vi "RTM - Import from XML.vi"(8 "error in (no error)":errorcluster, 11 "Node Ptr":u64 format="%.0x") -> (0 "error out":errorcluster)   [LabVIEW 2019, in "UDP-Custom-Device System Explorer.lvlib"]
uses:
  UDP-Custom-Device System Explorer.lvlib
panel:
  in  "Tag":string
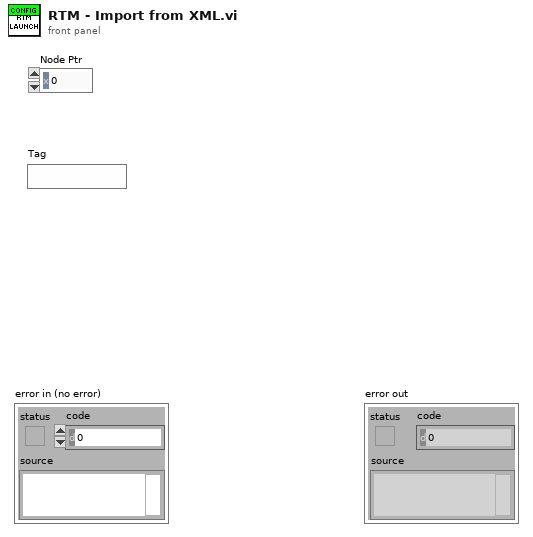
[diagram p1: front panel]
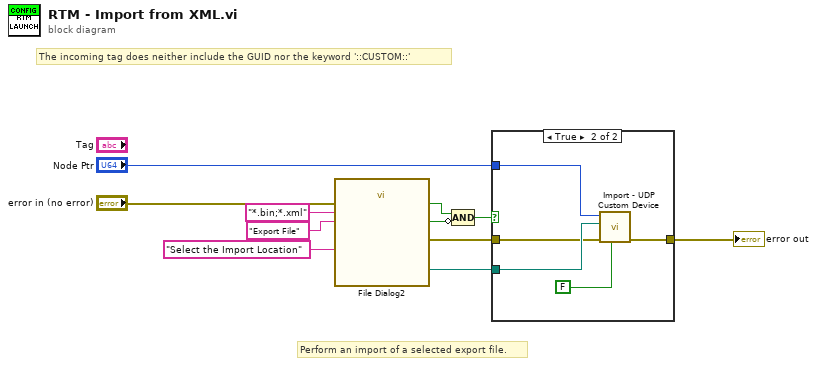
[diagram p0: block diagram]
diagram:
  # "Perform an import of a selected export file."
  # "The incoming tag does neither include the GUID nor the keyword '::CUSTOM::'"
  n1 = call "File Dialog2"("prompt"="Select the Import Location", "error in"="error in (no error)", "pattern (all files)"="*.bin;*.xml", "pattern label"="Export File") -> ("selected path"=w7:path, "exists"=w5:bool, "cancelled"=w4:bool, "error out"=w6:errorcluster)  [unwired: 8 in]
  n2 = Compound Arithmetic op=AND(w5, invert w4) -> (w3:bool)
  n3 = case shown="True" w3 {
    tunnel: w7 -> [_ w17]
    tunnel: w6 -> [w12 w16]
    tunnel: [w12 w15] -> w10
    tunnel: "Node Ptr" -> [_ w14]
    frame False {
    }
    frame True {
      n4 = call "Import - UDP Custom Device.vi"("New CD?"=FALSE, "error in (no error)"=w16, "Target File"=w17, "Device Item Ref in"=w14) -> ("error out"=w15:errorcluster)  [unwired: 7 in]
    }
  }
  "error out" <- w10
